vi "Print View Data Screen.vi"(6 "file names":string[](array[string]), 8 "Y Axis Names":string[](array[string]), 9 "X Axis Name":string, 11 "Graph Ref  in":refnum<vi>) -> ()   [LabVIEW 2019]
uses:
  Type Defs and Controls/Header Information.ctl
panel:
  out "name display":string[](array[string])
  out "Graph 3":cluster{dbl[], dbl[]}[](graph)
  out "Legend":string[](array[string])
  in  "Header Information in":T1
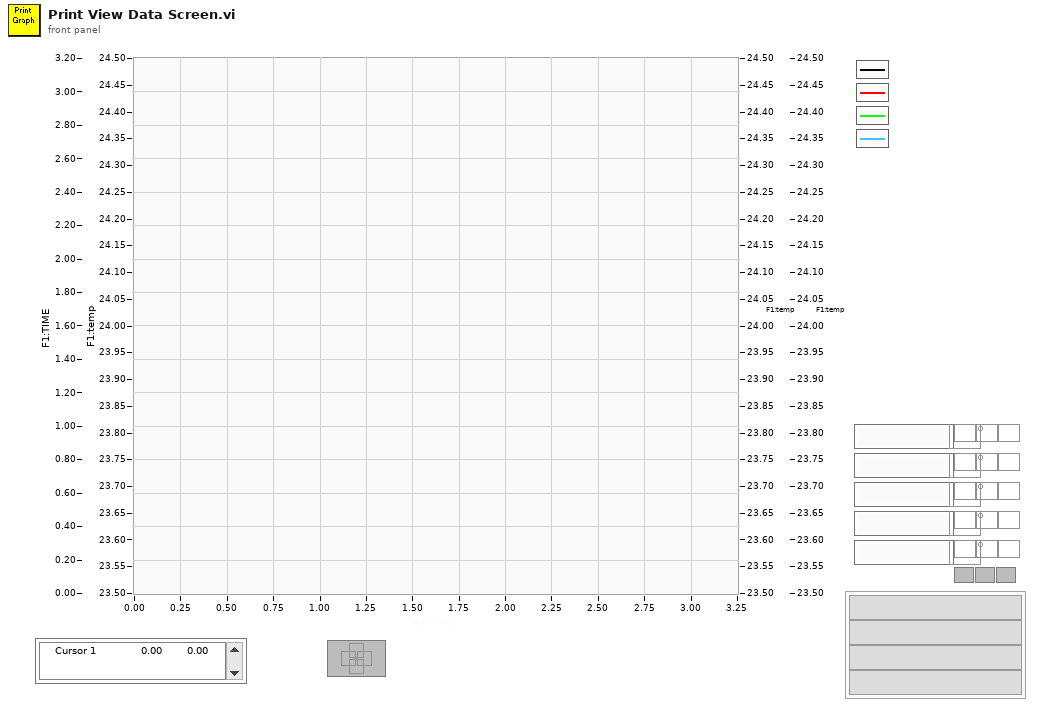
[diagram p1: front panel]
types:
  T1 = typedef "Header Information.ctl" = cluster{"TA Number":string, "Test Type":string, "Serial Number":string, "Comments":string}
  T2 = typedef "LVRangeTypeDef.ctl" = cluster{"Minimum":dbl, "Maximum":dbl, "Increment":dbl, "Minor Increment":dbl, "Start":dbl}
  T3 = typedef "LVPointDoubleTypeDef.ctl" = cluster{"Cursor X":dbl, "Cursor Y":dbl}
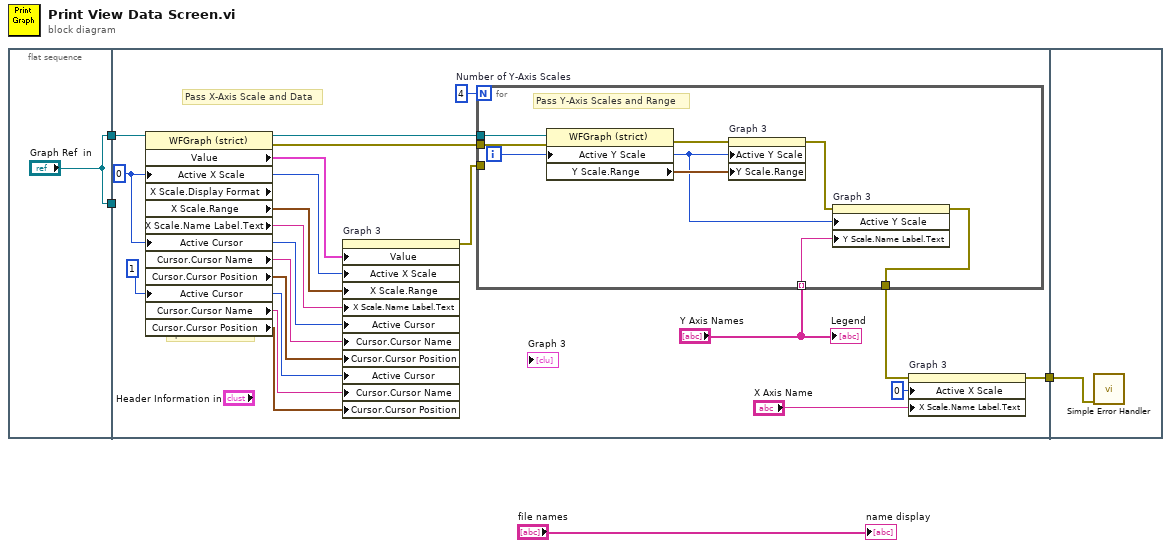
[diagram p0: block diagram]
diagram:
  n1 = flat-sequence {
    tunnel: ["Graph Ref  in"] -> w4
    tunnel: ["Graph Ref  in"] -> w3
    tunnel: w4 -> [w24]
    tunnel: w3 -> [_]
    tunnel: [w6] -> w2
    tunnel: w2 -> [w33]
    frame #0 {
    }
    frame #1 {
      w16 = 1 ("Active X Scale")
      w22 = 4  # Number of Y-Axis Scales
      w13 = 0 ("Active X Scale")
      # "Update Indicators"
      # "Pass X-Axis Scale and Data"
      n2 = property class="WFGraph (strict)" props=["Value", "Active X Scale", "X Scale", "Display Format", "X Scale", "Range", "X Scale", "Name Label", "Text", "Active Cursor", "Cursor", "Cursor Name", "Cursor", "Cursor Position", "Active Cursor", "Cursor", "Cursor Name", "Cursor", "Cursor Position"](reference=w24, "Active X Scale"=w13, "Active Cursor"=w13, "Active Cursor"=w16) -> (reference out=w23:refnum<vi>, error out=w11:errorcluster, "Value"=w21:cluster{dbl[], dbl[]}[], "X Scale.Range"=w20:T2, "X Scale.Name Label.Text"=w12:string, "Cursor.Cursor Name"=w18:string, "Cursor.Cursor Position"=w17:T3, "Cursor.Cursor Name"=w15:string, "Cursor.Cursor Position"=w14:T3)  [unwired: 1 in, 1 out]
      n3 = property on="Graph 3" class="XYGraph (strict)"("Value"=w21, "Active X Scale"=w13, "X Scale.Range"=w20, "X Scale.Name Label.Text"=w12, "Active Cursor"=w13, "Cursor.Cursor Name"=w18, "Cursor.Cursor Position"=w17, "Active Cursor"=w16, "Cursor.Cursor Name"=w15, "Cursor.Cursor Position"=w14) -> (error out=w19:errorcluster)  [unwired: 2 in, 1 out]
      n4 = for {
        N: w22 -> [_]
        tunnel: w23 -> [w32]
        tunnel: w19 -> [_]
        tunnel: w11 -> [w31]
        tunnel: "Y Axis Names" -> [w26] mode=indexing
        tunnel: [w25] -> w7
        i -> [w27]
        # "Pass Y-Axis Scales and Range"
        n5 = property class="WFGraph (strict)"(reference=w32, error in=w31, "Active Y Scale"=w27) -> (error out=w30:errorcluster, "Y Scale.Range"=w29:T2)  [unwired: 1 out]
        n6 = property on="Graph 3" class="XYGraph (strict)"(error in=w30, "Active Y Scale"=w27, "Y Scale.Range"=w29) -> (error out=w28:errorcluster)  [unwired: 1 in, 1 out]
        n7 = property on="Graph 3" class="XYGraph (strict)"(error in=w28, "Active Y Scale"=w27, "Y Scale.Name Label.Text"=w26) -> (error out=w25:errorcluster)  [unwired: 1 in, 1 out]
      }
      n8 = property on="Graph 3" class="XYGraph (strict)"(error in=w7, "Active X Scale"=0, "X Scale.Name Label.Text"="X Axis Name") -> (error out=w6:errorcluster)  [unwired: 1 in, 1 out]
      "Legend" <- "Y Axis Names"
    }
    frame #2 {
      n9 = call <vilib>:"Simple Error Handler.vi"("error in (no error)"=w33) -> ()  [unwired: 4 in, 5 out]
    }
  }
  "name display" <- "file names"
